vi "Resave_Normal_Dot-2.vi"(1 "starting index (dot)":i32, 2 "# column":i32, 3 "[IN] Source matrix":dbl[][](array[numeric]), 4 "[IN] Collect matrix":dbl[][](array[numeric])) -> (0 "[OUT] Collect matrix":dbl[][](array[numeric]))   [LabVIEW 2017]
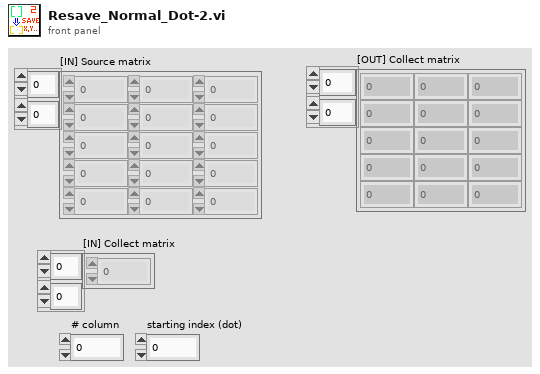
[diagram p1: front panel]
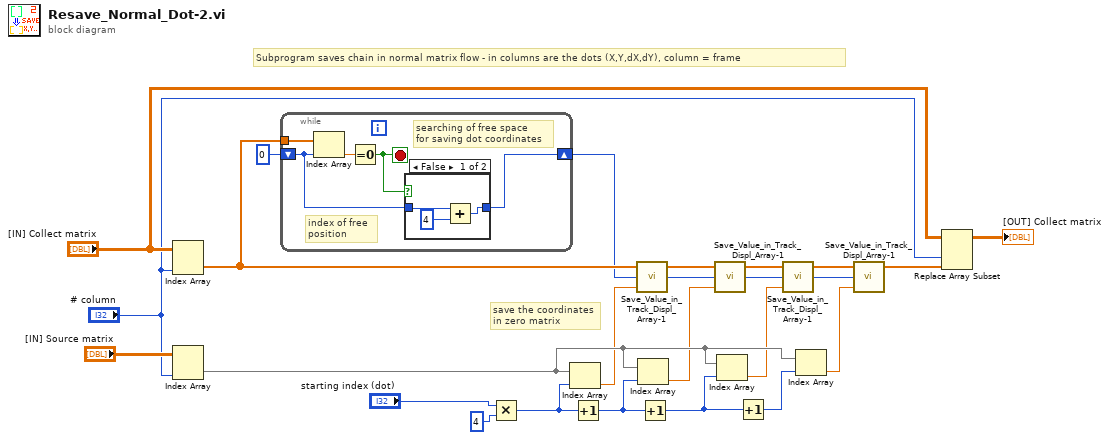
[diagram p0: block diagram]
diagram:
  # "Subprogram saves chain in normal matrix flow - in columns are the dots (X,Y,dX,dY), column = frame"
  # "save the coordinates\nin zero matrix"
  n1 = Index Array(array="[IN] Collect matrix", index (col)="# column") -> (element=w13:dbl[])  [unwired: 1 in]
  n2 = Index Array(array="[IN] Source matrix", index (col)="# column") -> (element=w22:dbl[])  [unwired: 1 in]
  n3 = while {
    tunnel: w13 -> [w30]
    shift-right: [w26] -> w12
    shift-left: 0 -> [w27]
    stop <- w28 stop-if-true
    # "index of free \nposition"
    # "searching of free space \nfor saving dot coordinates"
    n4 = Index Array(array=w30, index=w27) -> (element=w29:dbl)
    n5 = Equal To 0?(x=w29) -> (x = 0?=w28:bool)
    n6 = case shown="False" w28 {
      tunnel: w27 -> [w32 w34]
      tunnel: [w31 w34] -> w26
      frame False {
        n7 = Add(x=w32, y=4) -> (x+y=w31:i32)
      }
      frame True {
      }
    }
  }
  n8 = Multiply(x="starting index (dot)", y=4) -> (x*y=w14:i32)
  n9 = Index Array(array=w22, index=w14) -> (element=w11:dbl)
  n10 = Increment(x=w14) -> (x+1=w23:i32)
  n11 = call "Save_Value_in_Track_Displ_Array-1.vi"("[IN] Value"=w11, "[IN] Index"=w12, "[IN] Empty tracks\nfor points saving"=w13) -> ("[OUT] Index ++"=w9:i32, "[OUT Track with saved value"=w10:dbl[])  [unwired: 1 in]
  n12 = Index Array(array=w22, index=w23) -> (element=w8:dbl)
  n13 = Increment(x=w23) -> (x+1=w21:i32)
  n14 = call "Save_Value_in_Track_Displ_Array-1.vi"("[IN] Value"=w8, "[IN] Index"=w9, "[IN] Empty tracks\nfor points saving"=w10) -> ("[OUT] Index ++"=w6:i32, "[OUT Track with saved value"=w7:dbl[])  [unwired: 1 in]
  n15 = Index Array(array=w22, index=w21) -> (element=w5:dbl)
  n16 = Increment(x=w21) -> (x+1=w20:i32)
  n17 = call "Save_Value_in_Track_Displ_Array-1.vi"("[IN] Value"=w5, "[IN] Index"=w6, "[IN] Empty tracks\nfor points saving"=w7) -> ("[OUT] Index ++"=w3:i32, "[OUT Track with saved value"=w4:dbl[])  [unwired: 1 in]
  n18 = Index Array(array=w22, index=w20) -> (element=w2:dbl)
  n19 = call "Save_Value_in_Track_Displ_Array-1.vi"("[IN] Value"=w2, "[IN] Index"=w3, "[IN] Empty tracks\nfor points saving"=w4) -> ("[OUT Track with saved value"=w1:dbl[])  [unwired: 1 in, 1 out]
  n20 = Replace Array Subset(array="[IN] Collect matrix", new element=w1, index (col)="# column") -> (→"[OUT] Collect matrix":dbl[][])  [unwired: 1 in]
